vi "Initialize.vi"(8 "error in (no error)":errorcluster, 10 "DG Nr":i32, 11 "BME_DG_G02 in":refnum<class "BME_DG_G02.lvclass">) -> (0 "error out":errorcluster, 3 "BME_DG_G02 out":refnum<class "BME_DG_G02.lvclass">)   [LabVIEW 2009, in "BME_DG_G02.lvclass"]
uses:
  BME_DG_G02.lvclass
  BME_DG_G02_Chnl/BME_DG_G02_Chnl.lvclass
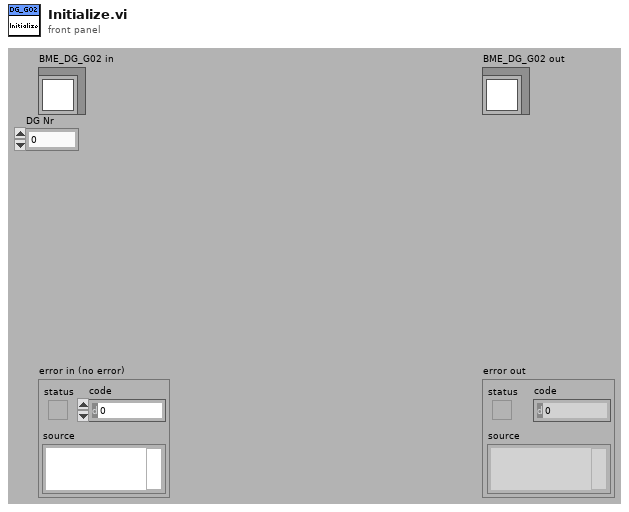
[diagram p1: front panel]
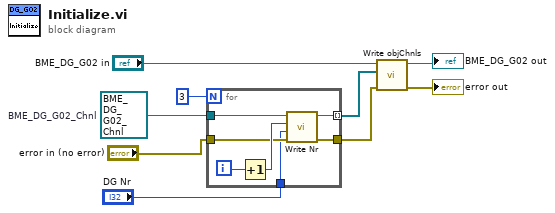
[diagram p0: block diagram]
diagram:
  w2 = refnum<class "BME_DG_G02_Chnl.lvclass"> refnum  # BME_DG_G02_Chnl
  n1 = for {
    N: 3 -> [_]
    tunnel: w2 -> [w15]
    tunnel: "error in (no error)" -> [w13]
    tunnel: [w12] -> w3
    tunnel: [w11] -> w4 mode=indexing
    tunnel: "DG Nr" -> [w10]
    i -> [w16]
    n2 = Increment(x=w16) -> (x+1=w14:i32)
    n3 = call-dynamic "Write Nr.vi"("error in (no error)"=w13, "DG Nr"=w10, "Nr"=w14, "BME_DG_Chnl in"=w15) -> ("error out"=w12:errorcluster, "BME_DG_Chnl out"=w11:refnum<class "BME_DG_G02_Chnl.lvclass">)  [unwired: 6 in]
  }
  n4 = call-dynamic "Write objChnls.vi"("error in (no error)"=w3, "objChnls"=w4, "BME_DG_Base in"="BME_DG_G02 in") -> ("error out"=→"error out":errorcluster, "BME_DG_Base out"=→"BME_DG_G02 out":refnum<class "BME_DG_G02.lvclass">)  [unwired: 7 in]
